vi "WriteMiscData.vi"(8 "error in (no error)":errorcluster) -> (0 "error out":errorcluster)   [LabVIEW 2018]
doc: "Put any data you want to log that doesn't fit elsewhere in this VI. This would be things like CPU Usage, Battery Voltage, etc."
uses:
  DataNames.ctl
  Framework/Robot Global Data.vi
  <vilib>/NI_Real-Time Target Support.lvlib
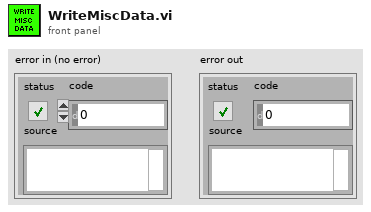
[diagram p1: front panel]
types:
  T1 = typedef "DataNames.ctl" = enum16{"RobotMode", "FMSConnected", "DriveLeft", "DriveRight", "EncoderLeft", "EncoderRight", "Angle", "LocationX", "LocationY", "CPU", "DriveOperation", "Battery"}
  T2 = typedef "NI_Real-Time Target Support.lvlib/RT CPU Load.ctl" = cluster{"Total (%)":dbl, "Time Critical (%)":dbl, "Timed Structures (%)":dbl, "High (%)":dbl, "Above Normal (%)":dbl, "Normal (%)":dbl, "Background (%)":dbl, "Idle (%)":dbl, "ISR (%)":dbl}
  T3 = typedef "WPI_DriverStationRobotMode2.ctl" = enum16{"Autonomous Disabled", "Autonomous Enabled", "Teleop Disabled", "Teleop Enabled", "Disconnected", "Finish", "Test Disabled", "Test Enabled", "Emergency Stopped"}
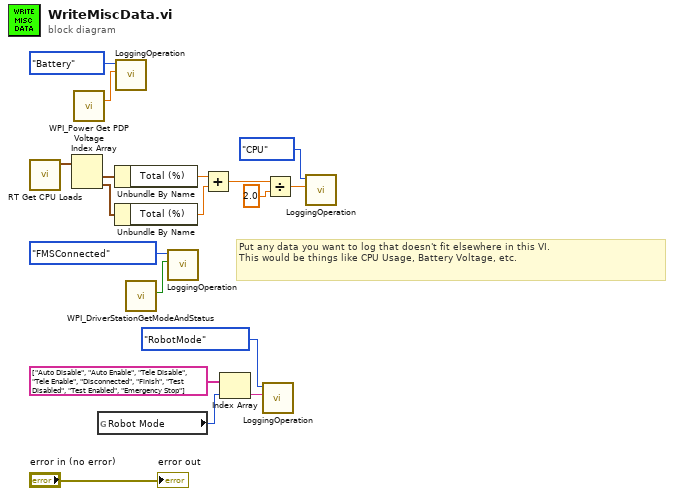
[diagram p0: block diagram]
diagram:
  # "Put any data you want to log that doesn't fit elsewhere in this VI.\nThis would be things like CPU Usage, Battery Voltage, etc."
  n1 = call <vilib>:"RT Get CPU Loads.vi"() -> ("CPU loads"=w4:T2[])  [unwired: 10 in, 1 out]
  n2 = Index Array(array=w4) -> (element #1=w3:T2, element #2=w2:T2)  [unwired: 2 in]
  n3 = call <vilib>:"WPI_Power Get PDP Voltage.vi"() -> ("voltage (V)"=w13:dbl)  [unwired: 14 in, 1 out]
  n4 = global read "Robot Global Data.vi" "Robot Mode"() -> (w7:T3)
  n5 = Unbundle By Name(w3) -> ("Total (%)"=w15:dbl)
  n6 = Unbundle By Name(w2) -> ("Total (%)"=w14:dbl)
  n7 = call "LoggingOperation.vi"("Data"=w13, "Name"=DataNames."Battery") -> ()  [unwired: 9 in, 1 out]
  n8 = call <vilib>:"WPI_DriverStationGetModeAndStatus.vi"() -> ("FMS Attached"=w6:bool)  [unwired: 10 in, 1 out]
  n9 = call "LoggingOperation.vi"("Data"=w6, "Name"=DataNames."FMSConnected") -> ()  [unwired: 9 in, 1 out]
  n10 = Add(x=w15, y=w14) -> (x+y=w16:dbl)
  n11 = Index Array(array=string[] ["Auto Disable", "Auto Enable", "Tele Disable", "Tele Enable", "Disconnected", "Finish", "Test Disabled", "Test Enabled", "Emergency Stop"], index=w7) -> (element=w5:string)
  n12 = call "LoggingOperation.vi"("Data"=w5, "Name"=DataNames."RobotMode") -> ()  [unwired: 9 in, 1 out]
  n13 = Divide(x=w16, y=2.0) -> (x/y=w18:dbl)
  n14 = call "LoggingOperation.vi"("Data"=w18, "Name"=DataNames."CPU") -> ()  [unwired: 9 in, 1 out]
  "error out" <- "error in (no error)"
